vi "coag pump volts.vi"(10 "mL/rev":dbl, 11 "coagulant flow [mL/s]":dbl) -> (0 "In Range?":bool, 1 "V":dbl, 3 "rpm":dbl)   [LabVIEW 2015]
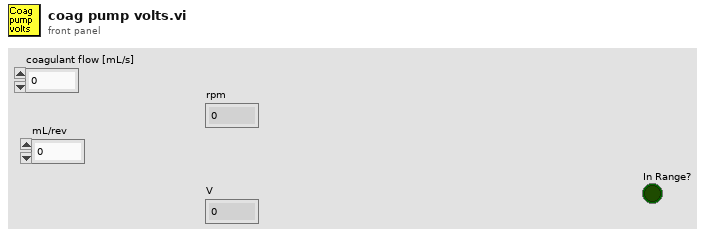
[diagram p1: front panel]
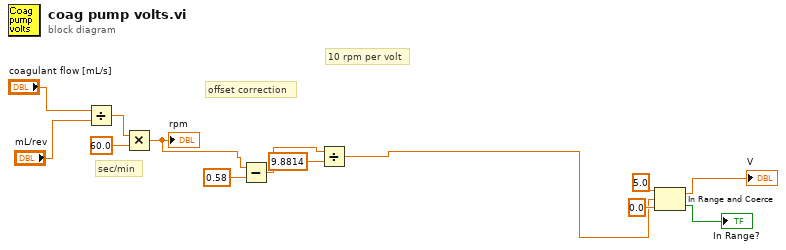
[diagram p0: block diagram]
diagram:
  # "10 rpm per volt"
  # "offset correction"
  # "sec/min"
  n1 = Divide(x="coagulant flow [mL/s]", y="mL/rev") -> (x/y=w11:dbl)
  n2 = Multiply(x=w11, y=60.0) -> (x*y=w3:dbl)
  "rpm" <- w3
  n3 = Subtract(x=w3, y=0.58) -> (x-y=w2:dbl)
  n4 = Divide(x=w2, y=9.8814) -> (x/y=w1:dbl)
  n5 = In Range and Coerce(upper limit=5.0 ("x"), x=w1, lower limit=0.0) -> (coerced(x)=→"V":dbl, In Range?=→"In Range?":bool)
